vi "number5-sub2.vi"(4 "Numeric":i32, 5 "Numeric 2":i32, 7 "array":i32[][](array[numeric])) -> (3 "array 2":i32[][](array[numeric]))   [LabVIEW 2014]
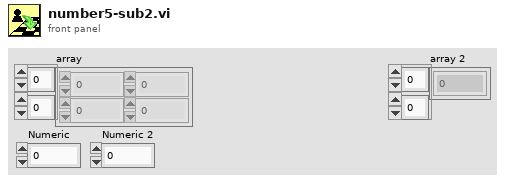
[diagram p1: front panel]
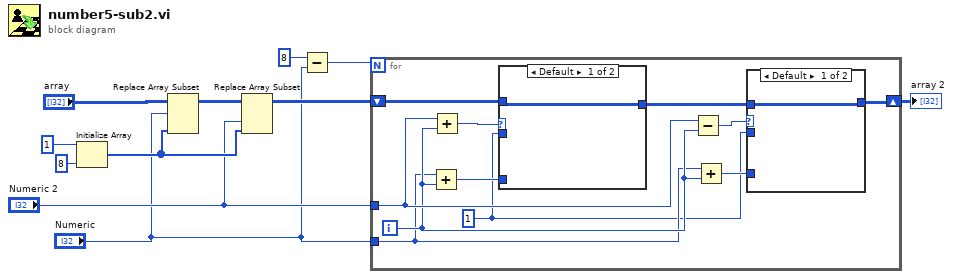
[diagram p0: block diagram]
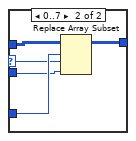
[diagram p2: hidden frame]
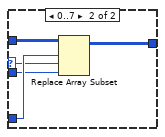
[diagram p3: hidden frame]
diagram:
  n1 = Initialize Array(1 ("element"), 8 ("dimension size")) -> (w7:i32[])
  n2 = Replace Array Subset(array="array", new element=w7, index (row)="Numeric") -> (w10:i32[][])  [unwired: 1 in]
  n3 = Replace Array Subset(array=w10, new element=w7, index (col)="Numeric 2") -> (w4:i32[][])  [unwired: 1 in]
  n4 = Subtract(x=8, y="Numeric") -> (x-y=w6:i32)
  n5 = for {
    N: w6 -> [_]
    shift-right: [w12] -> w1
    shift-left: w4 -> [w17]
    tunnel: "Numeric 2" -> [w21]
    tunnel: "Numeric" -> [w19]
    i -> [w20]
    w14 = 1 ("new element/subarray")
    n6 = Add(x=w19, y=w20) -> (x+y=w18:i32)
    n7 = Add(x=w21, y=w20) -> (x+y=w22:i32)
    n8 = case shown="Default" w22 {
      selector: w22 -> [_ w31]
      tunnel: w18 -> [_ w32]
      tunnel: w17 -> [w29 w34]
      tunnel: [w29 w33] -> w13
      tunnel: w14 -> [_ w30]
      frame Default {
      }
      frame 0..7 {
        n9 = Replace Array Subset(array=w34, new element=w30, index (row)=w32, index (col)=w31) -> (w33:i32[][])
      }
    }
    n10 = Subtract(x=w21, y=w20) -> (x-y=w16:i32)
    n11 = Add(x=w19, y=w20) -> (x+y=w15:i32)
    n12 = case shown="Default" w16 {
      selector: w16 -> [_ w25]
      tunnel: w15 -> [_ w26]
      tunnel: w14 -> [_ w24]
      tunnel: w13 -> [w23 w28]
      tunnel: [w23 w27] -> w12
      frame Default {
      }
      frame 0..7 {
        n13 = Replace Array Subset(array=w28, new element=w24, index (row)=w26, index (col)=w25) -> (w27:i32[][])
      }
    }
  }
  "array 2" <- w1
